vi "AlliGator Get Local Fit Results String.vi"(6 "Parameters SDV":dbl[](array[numeric]), 7 "Decay Sum":dbl, 8 "Parameters":dbl[](array[numeric]), 9 "Y":i32, 10 "X":i32, 11 "[Decay Fit Parameter Name]":T1[](array[typedef])) -> (3 "Fit Results String":string)   [LabVIEW 2021, in "AlliGator Decay Fit Parameter Map.lvlib"]
doc: "Builds Decay Fit Parmeters string."
uses:
  AlliGator Decay Fit Parameter Map.lvlib
  Fits/IRF(X)PSED/Decay Fit Parameters & Derived Quantities List v2.ctl
  Fits/Fits.lvlib
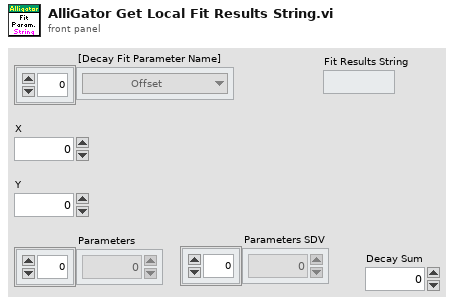
[diagram p1: front panel]
types:
  T1 = typedef "Fits.lvlib/Decay Fit Parameters & Derived Quantities List v2.ctl" = enum16{"Offset", "Baseline", "A_1", "tau_1", "A_2", "tau_2", "<tau>_a", "f1_a", "f2_a", "<tau>_i", "f1_i", "f2_i", "-", "R^2", "Chi^2"}
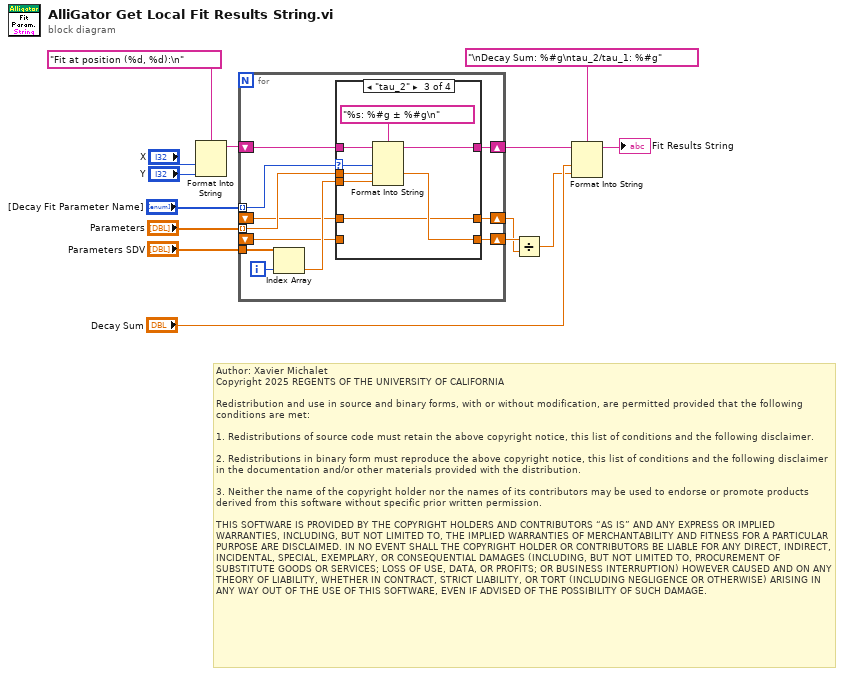
[diagram p0: block diagram]
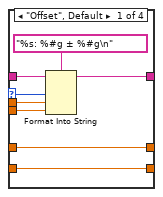
[diagram p2: hidden frame]
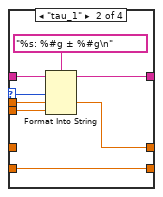
[diagram p3: hidden frame]
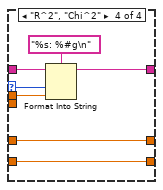
[diagram p4: hidden frame]
diagram:
  # "Author: Xavier Michalet\nCopyright 2025 REGENTS OF THE UNIVERSITY OF CALIFORNIA\n\nRedistribution and use in source and binary forms, with or without modification, are permitted provided that the following conditions are met:\n\n1. Redistributions of source code must retain the above copyright notice, this list of conditions and the following disclaimer.\n\n2. Redistributions in binary form must reproduce the above copyright notice, this list of conditions and the following disclaimer in the documentation and/or other materials provided with the distribution.\n\n3. Neither the name of the copyright holder nor the names of its contributors may be used to endorse or promote products derived from this software without specific prior written permission.\n\nTHIS SOFTWARE IS PROVIDED BY THE COPYRIGHT HOLDERS AND CONTRIBUTORS “AS IS” AND ANY EXPRESS OR IMPLIED WARRANTIES, INCLUDING, BUT NOT LIMITED TO, THE IMPLIED WARRANTIES OF MERCHANTABILITY AND FITNESS FOR A PARTICULAR PURPOSE ARE DISCLAIMED. IN NO EVENT SHALL THE COPYRIGHT HOLDER OR CONTRIBUTORS BE LIABLE FOR ANY DIRECT, INDIRECT, INCIDENTAL, SPECIAL, EXEMPLARY, OR CONSEQUENTIAL DAMAGES (INCLUDING, BUT NOT LIMITED TO, PROCUREMENT OF SUBSTITUTE GOODS OR SERVICES; LOSS OF USE, DATA, OR PROFITS; OR BUSINESS INTERRUPTION) HOWEVER CAUSED AND ON ANY THEORY OF LIABILITY, WHETHER IN CONTRACT, STRICT LIABILITY, OR TORT (INCLUDING NEGLIGENCE OR OTHERWISE) ARISING IN ANY WAY OUT OF THE USE OF THIS SOFTWARE, EVEN IF ADVISED OF THE POSSIBILITY OF SUCH DAMAGE."
  n1 = Format Into String(format string="Fit at position (%d, %d):\n", "X", "Y") -> (resulting string=w11:string)  [unwired: 2 in, 1 out]
  n2 = for {
    shift-right: [w24] -> w8
    shift-left: w11 -> [w25]
    tunnel: "[Decay Fit Parameter Name]" -> [w23] mode=indexing
    tunnel: "Parameters" -> [w22] mode=indexing
    tunnel: "Parameters SDV" -> [w21]
    shift-right: [w18] -> w2
    shift-left: _ -> [w16]
    shift-right: [w17] -> w3
    shift-left: _ -> [w15]
    i -> [w20]
    n3 = Index Array(array=w21, index=w20) -> (element=w19:dbl)
    n4 = case shown="\"tau_2\"" w23 {
      selector: w23 -> [w31 w38 w45 w52]
      tunnel: w25 -> [w33 w40 w47 w54]
      tunnel: [w32 w39 w46 w53] -> w24
      tunnel: w22 -> [w30 w35 w42 w51]
      tunnel: w19 -> [w29 w37 w44 _]
      tunnel: [w27 w35 w41 w49] -> w18
      tunnel: [w26 w34 w42 w48] -> w17
      tunnel: w16 -> [w27 _ w41 w49]
      tunnel: w15 -> [w26 w34 _ w48]
      frame "Offset", Default {
        n5 = Format Into String(format string="%s: %#g ± %#g\n", initial string=w33, w31, w30, w29) -> (resulting string=w32:string)  [unwired: 1 in, 1 out]
      }
      frame "tau_1" {
        n6 = Format Into String(format string="%s: %#g ± %#g\n", initial string=w40, w38, w35, w37) -> (resulting string=w39:string)  [unwired: 1 in, 1 out]
      }
      frame "tau_2" {
        n7 = Format Into String(format string="%s: %#g ± %#g\n", initial string=w47, w45, w42, w44) -> (resulting string=w46:string)  [unwired: 1 in, 1 out]
      }
      frame "R^2", "Chi^2" {
        n8 = Format Into String(format string="%s: %#g\n", initial string=w54, w52, w51) -> (resulting string=w53:string)  [unwired: 1 in, 1 out]
      }
    }
  }
  n9 = Divide(x=w3, y=w2) -> (x/y=w1:dbl)
  n10 = Format Into String(format string="\nDecay Sum: %#g\ntau_2/tau_1: %#g", initial string=w8, "Decay Sum", w1) -> (resulting string=→"Fit Results String":string)  [unwired: 1 in, 1 out]
